vi "lua_xmove.vi"(8 "error in (no error)":errorcluster, 9 "n":i32, 10 "to lua_state_p":u64, 11 "from lua_state_p":u64) -> (0 "error out":errorcluster, 2 "to lua_state_p out":u64, 3 "from lua_state_p out":u64)   [LabVIEW 2020, in "lua.dll.lvlib"]
doc: "Exchange values between different threads of the same state.\n\nThis function pops n values from the stack from, and pushes them onto the stack to."
uses:
  lua.dll.lvlib
  lua54.dll
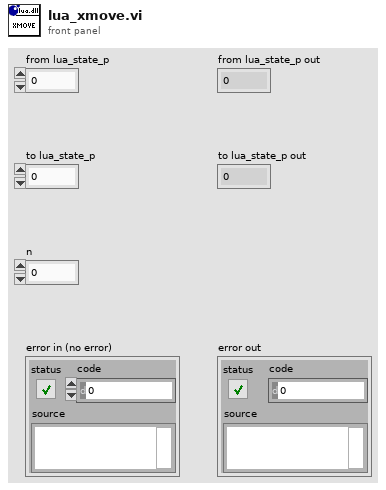
[diagram p1: front panel]
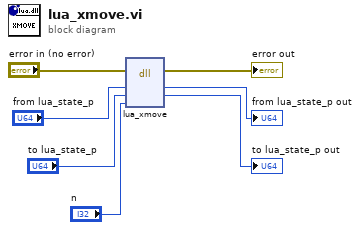
[diagram p0: block diagram]
diagram:
  n1 = dll-call lib="C:/Users/Nicholas Folse/Documents/workspace/github-tauterra.llc/Lua for LabVIEW/lib/lua.dll/lua54**.*" fn="lua_xmove"(error in="error in (no error)", "from lua_state_p"="from lua_state_p", "to lua_state_p"="to lua_state_p", "n"="n") -> (error out=→"error out":errorcluster, "from lua_state_p"=→"from lua_state_p out":u64, "to lua_state_p"=→"to lua_state_p out":u64)  [unwired: 4 in, 1 out]
